vi "Main.vi"() -> ()   [LabVIEW 2020]
doc: "This template is for the Queued Message Handler design pattern.\n\nThe Event Handling Loop generates messages based on user interface actions.\n\nThe Message Handling Loop processes messages generated by the Event Handling Loop, or by other messages. The messages are string values, so new messages can be added easily to the Message Cases case structure in the Message Handling Loop. Each message cluster can also provide an optional value for Message Data, which is a variant that can be converted to whatever message-specific data is required."
uses:
  controls/UI Data.ctl
  <vilib>/Instr/_visa.llb/VISA Configure Serial Port (Instr).vi
  support/Message Queue/Enqueue Message (Single).vi
  <vilib>/Utility/error.llb/Error Cluster From Error Code.vi
  <vilib>/ErrorRing/Error Ring.xnode
  support/Message Queue/Message Queue.lvlib
  support/User Event - Stop/User Event - Stop.lvlib
panel:
  in  "Porta":refnum<visa-resource-name>
  in  "Atualizar":bool
  in  "Azul":u8(slide) scale=0.0..255.0
  in  "Verde":u8(slide) scale=0.0..255.0
  in  "Vermelho":u8(slide) scale=0.0..255.0
  in  "Brilho":u8(slide) scale=0.0..255.0
  out "Saida":string
  in  "Exit":bool
  # "Controle de Cores"
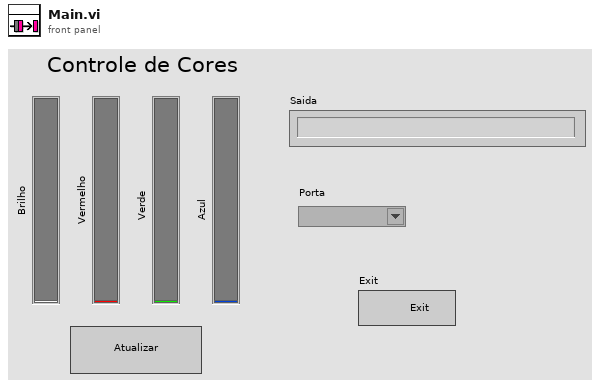
[diagram p1: front panel]
types:
  T1 = typedef "UI Data.ctl" = cluster{"Boolean <Replace Me>":bool, "String <Replace Me>":string, "Numeric <Replace Me>":dbl, "Do Something Ref":refnum<vi>, "Do Something Else Ref":refnum<vi>, "Data Display Ref":refnum<vi>, "Exit Button Ref":refnum<vi>}
  T2 = typedef "Message Queue.lvlib/All Message Queues.ctl" = cluster{"UI":refnum<queue>}
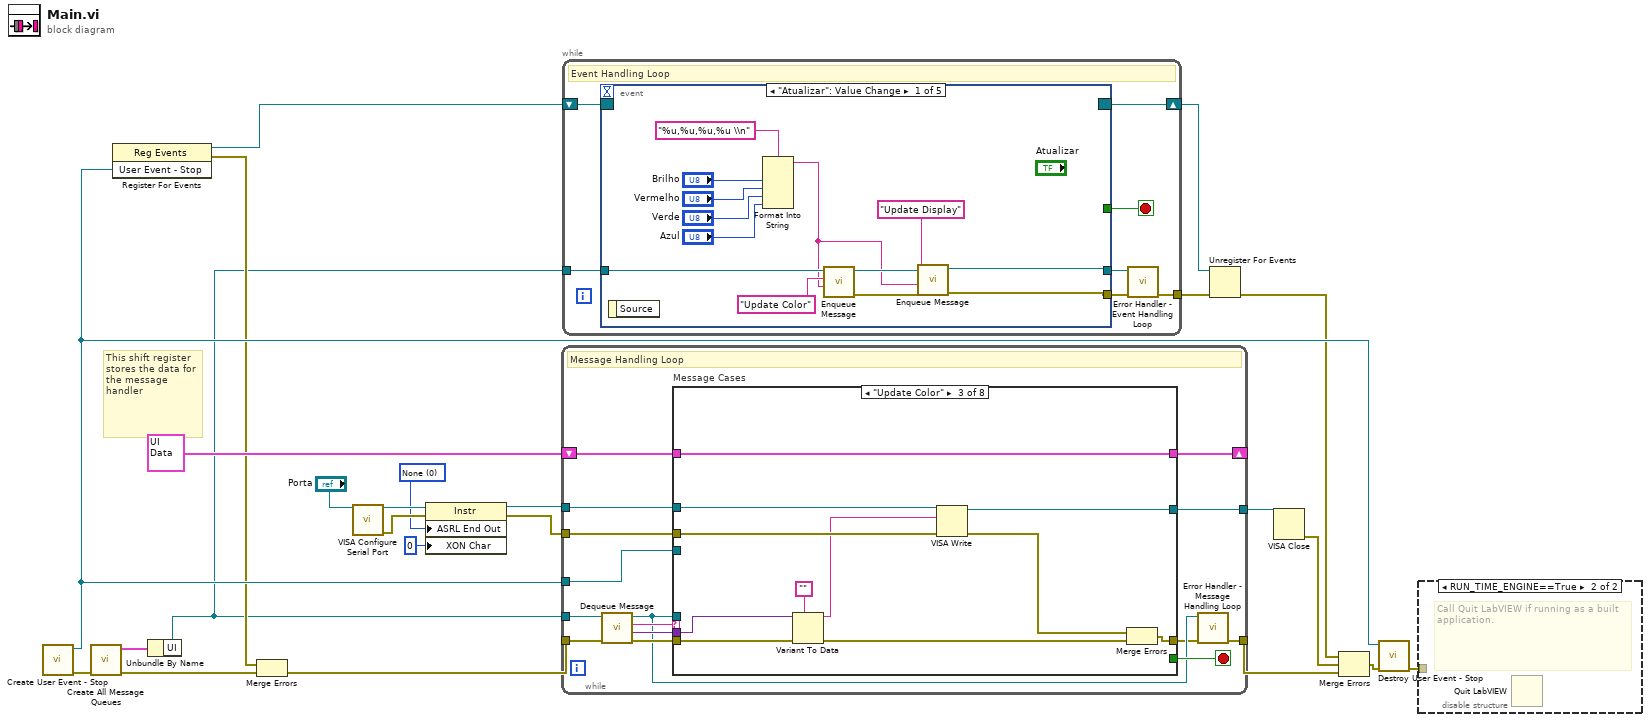
[diagram p0: block diagram]
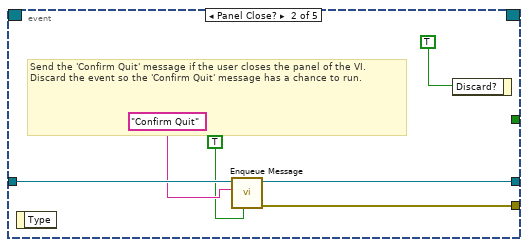
[diagram p3: hidden frame]
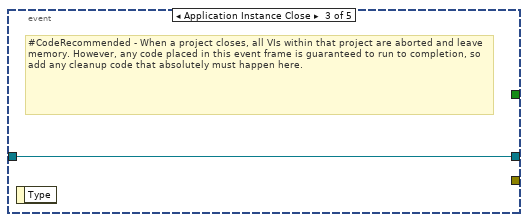
[diagram p4: hidden frame]
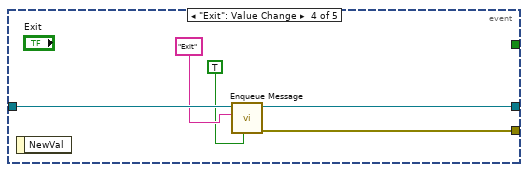
[diagram p5: hidden frame]
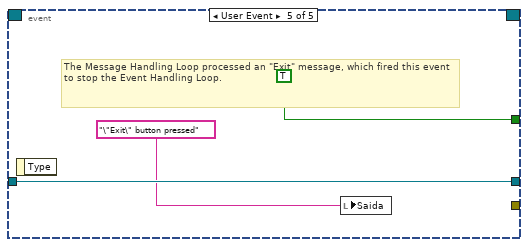
[diagram p6: hidden frame]
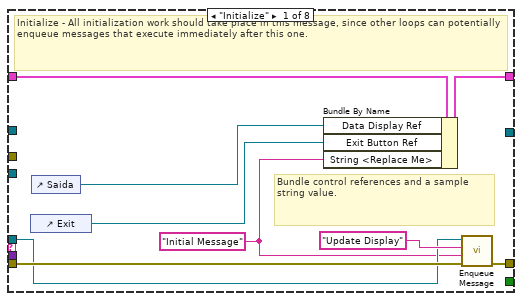
[diagram p7: hidden frame]
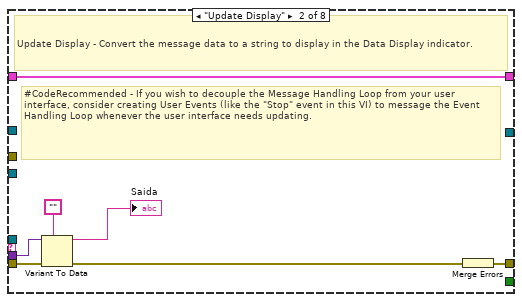
[diagram p8: hidden frame]
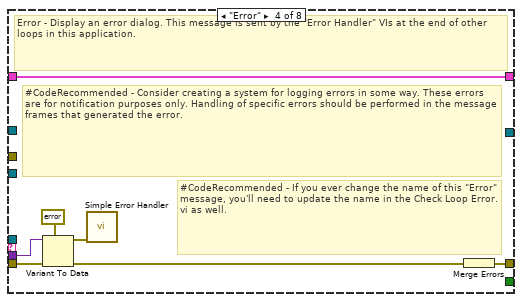
[diagram p9: hidden frame]
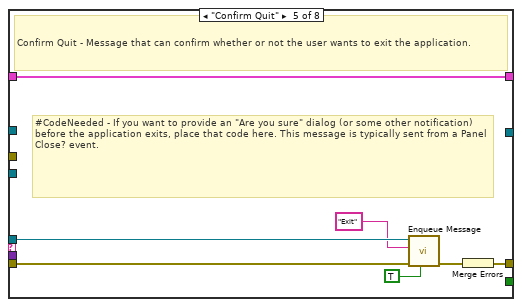
[diagram p10: hidden frame]
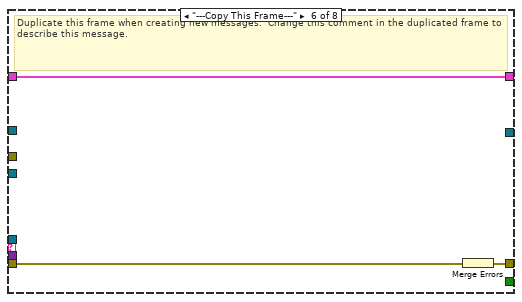
[diagram p11: hidden frame]
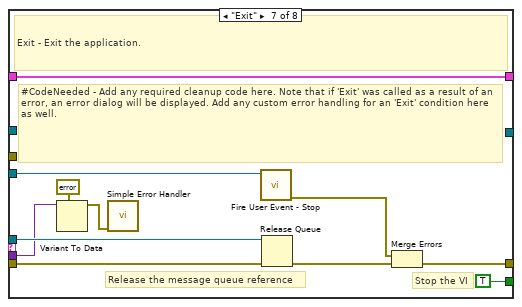
[diagram p12: hidden frame]
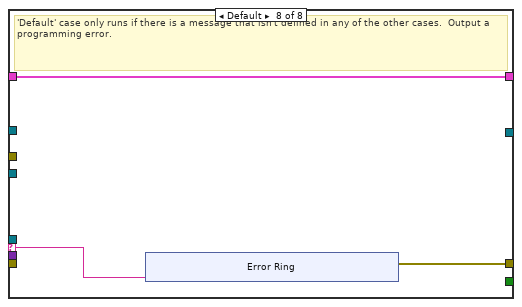
[diagram p13: hidden frame]
diagram:
  w2 = u16 0 items=["None", "Last Bit", "TermChar", "Break"] ("Serial Settings:End Mode for Writes")
  # "This shift register stores the data for the message handler"
  n1 = call "Create User Event - Stop.vi"() -> ("error out"=w21:errorcluster, "User Event - Stop"=w14:refnum<user-event>)  [unwired: 10 in]
  n2 = call "Create All Message Queues.vi"("error in (no error)"=w21) -> ("error out"=w24:errorcluster, "Message Queues out"=w23:T2)  [unwired: 9 in]
  n3 = register-events(w14) -> (reference out=w15:refnum<event-registration>, error out=w12:errorcluster)  [unwired: 2 in]
  n4 = Unbundle By Name(w23) -> ("UI"=w3:refnum<queue>)
  n5 = Merge Errors(w12, w24) -> (w13:errorcluster)
  n6 = call-poly "VISA Configure Serial Port"("VISA resource name"="Porta") -> ("VISA resource name out"=w7:refnum<visa-resource-name>, "error out"=w5:errorcluster)  [unwired: 13 in]
  n7 = property class="Instr"(reference=w7, error in=w5, "ASRL End Out"=w2, "XON Char"=u8 0 ("Serial Settings:Flow Control XON Character")) -> (reference out=w6:refnum<visa-resource-name>, error out=w4:errorcluster)
  n8 = while {
    tunnel: w3 -> [w31]
    shift-right: [w38] -> _
    shift-left: T1 {"Boolean <Replace Me>"=FALSE, "String <Replace Me>"="", "Numeric <Replace Me>"=0.0, "Do Something Ref"=refnum, "Do Something Else Ref"=refnum, "Data Display Ref"=refnum, "Exit Button Ref"=refnum} ("Data Cluster") -> [w39]
    tunnel: w14 -> [w36]
    tunnel: w13 -> [w35]
    tunnel: [w29] -> w22
    tunnel: w4 -> [w27]
    tunnel: w6 -> [w26]
    tunnel: [w25] -> w9
    stop <- w37 stop-if-true
    # "Message Handling Loop"
    n9 = call "Dequeue Message.vi"("error in (no error)"=w35, "Message Queue"=w31) -> ("error out"=w34:errorcluster, "Message Data"=w32:variant, "Message"=w33:string, "dup Message Queue"=w30:refnum<queue>)  [unwired: 6 in]
    n10 = case "Message Cases" shown="\"Update Color\"" w33 {
      selector: w33 -> [_ _ _ _ _ _ _ w95]
      tunnel: w30 -> [w41 _ _ _ w76 _ w94 _]
      tunnel: w34 -> [w47 w53 w64 w73 w80 w83 w87 _]
      tunnel: [w48 w54 w65 w67 w78 w81 w90 w96] -> w28
      tunnel: w39 -> [w46 w55 w66 w72 w79 w82 w93 w97]
      tunnel: [w45 w55 w66 w72 w79 w82 w93 w97] -> w38
      tunnel: [_ _ _ _ _ _ TRUE _] -> w37
      tunnel: w32 -> [_ w52 w63 w71 _ _ w84 _]
      tunnel: w36 -> [_ _ _ _ _ _ w89 _]
      tunnel: w27 -> [_ _ w60 _ _ _ _ _]
      tunnel: w26 -> [_ _ w59 _ _ _ _ _]
      tunnel: [_ _ w58 _ _ _ _ _] -> w25
      frame "Initialize" {
        w40 = "Initial Message" ("Initial Message")
        # "Bundle control references and a sample string value."
        # "Initialize - All initialization work should take place in this message, since other loops can potentially enqueue messages that execute immediately after this one."
        n11 = control-ref of="Exit"() -> (w43:refnum<vi>)
        n12 = control-ref of="Saida"() -> (w44:refnum<vi>)
        n13 = Bundle By Name(cluster=w46, "Data Display Ref"=w44, "Exit Button Ref"=w43, "String <Replace Me>"=w40) -> (w45:T1)
        n14 = call-poly "Enqueue Message.vi"("error in (no error)"=w47, "Message Data"=w40, "Message"="Update Display", "Message Queue"=w41) -> ("error out"=w48:errorcluster)  [unwired: 6 in, 1 out]
      }
      frame "Update Display" {
        # "#CodeRecommended - If you wish to decouple the Message Handling Loop from your user interface, consider creating User Events (like the \"Stop\" event in this VI) to message the Event Handling Loop whenever the user interface needs updating."
        # "Update Display - Convert the message data to a string to display in the Data Display indicator."
        n15 = Variant To Data(error in=w53, type="", Variant=w52) -> (data=→"Saida":string, error out=w50:errorcluster)
        n16 = Merge Errors(w50) -> (w54:errorcluster)
      }
      frame "Update Color" {
        n17 = Variant To Data(error in=w64, type="", Variant=w63) -> (data=w56:string, error out=w61:errorcluster)
        n18 = VISA Write(VISA resource name=w59, write buffer=w56, error in (no error)=w60) -> (VISA resource name out=w58:refnum<visa-resource-name>, error out=w57:errorcluster)  [unwired: 1 out]
        n19 = Merge Errors(w57, w61) -> (w65:errorcluster)
      }
      frame "Error" {
        # "#CodeRecommended - If you ever change the name of this \"Error\" message, you'll need to update the name in the Check Loop Error.vi as well."
        # "#CodeRecommended - Consider creating a system for logging errors in some way. These errors are for notification purposes only. Handling of specific errors should be performed in the message frames that generated the error."
        # "Error - Display an error dialog. This message is sent by the \"Error Handler\" VIs at the end of other loops in this application."
        n20 = Variant To Data(error in=w73, type=errorcluster {"status"=FALSE, "code"=0, "source"=""} ("error constant"), Variant=w71) -> (data=w69:errorcluster, error out=w68:errorcluster)
        n21 = call <vilib>:"Simple Error Handler.vi"("error in (no error)"=w69) -> ()  [unwired: 4 in, 5 out]
        n22 = Merge Errors(w68) -> (w67:errorcluster)
      }
      frame "Confirm Quit" {
        # "#CodeNeeded - If you want to provide an \"Are you sure\" dialog (or some other notification) before the application exits, place that code here. This message is typically sent from a Panel Close? event."
        # "Confirm Quit - Message that can confirm whether or not the user wants to exit the application."
        n23 = call-poly "Enqueue Message.vi"("Priority Message? (F)"=TRUE, "error in (no error)"=w80, "Message"="Exit", "Message Queue"=w76) -> ("error out"=w77:errorcluster)  [unwired: 6 in, 1 out]
        n24 = Merge Errors(w77) -> (w78:errorcluster)
      }
      frame "---Copy This Frame---" {
        # "Duplicate this frame when creating new messages.  Change this comment in the duplicated frame to describe this message."
        n25 = Merge Errors(w83) -> (w81:errorcluster)
      }
      frame "Exit" {
        # "Stop the VI"
        # "Release the message queue reference"
        # "#CodeNeeded - Add any required cleanup code here. Note that if 'Exit' was called as a result of an error, an error dialog will be displayed. Add any custom error handling for an 'Exit' condition here as well."
        # "Exit - Exit the application."
        n26 = Variant To Data(type=errorcluster {"status"=FALSE, "code"=0, "source"=""} ("error constant"), Variant=w84) -> (data=w85:errorcluster)  [unwired: 1 in, 1 out]
        n27 = call <vilib>:"Simple Error Handler.vi"("error in (no error)"=w85) -> ()  [unwired: 4 in, 5 out]
        n28 = call "Fire User Event - Stop.vi"("User Event - Stop"=w89) -> ("error out"=w88:errorcluster)  [unwired: 10 in]
        n29 = Release Queue(queue=w94, error in (no error)=w87) -> (error out=w91:errorcluster)  [unwired: 1 in, 2 out]
        n30 = Merge Errors(w88, w91) -> (w90:errorcluster)
      }
      frame Default {
        # "'Default' case only runs if there is a message that isn't defined in any of the other cases.  Output a programming error."
        n31 = xnode "Error Ring"("parameter 0"=w95) -> ("error out"=w96:errorcluster)
      }
    }
    n32 = call "Error Handler - Message Handling Loop.vi"("error in (no error)"=w28, "Message Queue"=w30) -> ("dup error in"=w29:errorcluster)  [unwired: 8 in, 1 out]
  }
  n33 = while {
    tunnel: w3 -> [w111]
    shift-right: [w109] -> w19
    shift-left: w15 -> [w110]
    tunnel: [w105] -> w16
    stop <- w107 stop-if-true
    # "Event Handling Loop"
    n34 = event shown="[0] \"Atualizar\": Value Change" {
      selector: w110 -> [_ _ _ _ _]
      dyn-events: [_ _ _ _ _] -> w109
      timeout: _ -> [_ _ _ _ _]
      tunnel: [_ _ _ _ TRUE ("Discard?")] -> w107
      tunnel: w111 -> [w124 w129 w131 w136 w139]
      tunnel: [w114 w128 _ w135 _] -> w108
      tunnel: [w116 w127 w131 w134 w139] -> w106
      event "Atualizar": Value Change {
        n35 = event-data() -> ()  [unwired: 1 in, 1 out]
        n36 = Format Into String(format string="%u,%u,%u,%u \\n", "Brilho", "Vermelho", "Verde", "Azul") -> (resulting string=w113:string)  [unwired: 2 in, 1 out]
        n37 = call-poly "Enqueue Message.vi"("Message Data"=w113, "Message"="Update Color", "Message Queue"=w124) -> ("error out"=w115:errorcluster, "dup Message Queue"=w117:refnum<queue>)  [unwired: 7 in]
        n38 = call-poly "Enqueue Message.vi"("error in (no error)"=w115, "Message Data"=w113, "Message"="Update Display", "Message Queue"=w117) -> ("error out"=w114:errorcluster, "dup Message Queue"=w116:refnum<queue>)  [unwired: 6 in]
      }
      event Panel Close? {
        # "Send the 'Confirm Quit' message if the user closes the panel of the VI. Discard the event so the 'Confirm Quit' message has a chance to run."
        n39 = event-data() -> ()  [unwired: 1 in, 1 out]
        n40 = call-poly "Enqueue Message.vi"("Priority Message? (F)"=TRUE, "Message"="Confirm Quit", "Message Queue"=w129) -> ("error out"=w128:errorcluster, "dup Message Queue"=w127:refnum<queue>)  [unwired: 7 in]
        n41 = event-data("Discard?"=TRUE) -> ()  [unwired: 1 in, 1 out]
      }
      event Application Instance Close {
        # "#CodeRecommended - When a project closes, all VIs within that project are aborted and leave memory. However, any code placed in this event frame is guaranteed to run to completion, so add any cleanup code that absolutely must happen here."
        n42 = event-data() -> ()  [unwired: 1 in, 1 out]
      }
      event "Exit": Value Change {
        n43 = event-data() -> ()  [unwired: 1 in, 1 out]
        n44 = call-poly "Enqueue Message.vi"("Priority Message? (F)"=TRUE, "Message"="Exit", "Message Queue"=w136) -> ("error out"=w135:errorcluster, "dup Message Queue"=w134:refnum<queue>)  [unwired: 7 in]
      }
      event User Event {
        # "The Message Handling Loop processed an \"Exit\" message, which fired this event to stop the Event Handling Loop."
        n45 = event-data() -> ()  [unwired: 1 in, 1 out]
        n46 = local write "Saida"("\"Exit\" button pressed" ("VI Stopped")) -> ()
      }
    }
    n47 = call "Error Handler - Event Handling Loop.vi"("error in (no error)"=w108, "Message Queue"=w106) -> ("dup error in"=w105:errorcluster)  [unwired: 8 in, 1 out]
  }
  n48 = Unregister For Events(event registration refnum=w19, error in=w16) -> (error out=w11:errorcluster)
  n49 = VISA Close(VISA resource name=w9) -> (error out=w10:errorcluster)  [unwired: 1 in]
  n50 = Merge Errors(w11, w10, w22) -> (w20:errorcluster)
  n51 = call "Destroy User Event - Stop.vi"("error in (no error)"=w20, "User Event - Stop"=w14) -> ("error out"=w17:errorcluster)  [unwired: 9 in]
  n52 = disable-structure shown="RUN_TIME_ENGINE==True" {
    disable-tunnel: w17 -> [_ _]
    frame condition #0 (active) {
    }
    frame condition #1 {
      # "Call Quit LabVIEW if running as a built application."
      n53 = Quit LabVIEW() -> ()  [unwired: 1 in]
    }
  }
